vi "用户信息.vi"() -> ()   [LabVIEW 2020]
panel:
  out "用户信息":T1
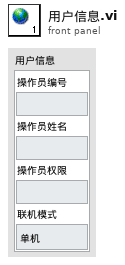
[diagram p1: front panel]
types:
  T1 = cluster{"操作员编号":string, "操作员姓名":string, "操作员权限":string, "联机模式":enum16{"单机", "追溯"}}
diagram:
